vi "Generate_WayPoints_Hopping WITH VariablePauseTIME.vi"(11 "Input Cluster":T2={"Scan Rate (um/s)"=15.0, "X Start"=15.0, "X End"=15.0, "Y Start"=15.0, "Y End"=15.0, " Z Start"=15.0, "HoppingDistance"=1.0, "V"=15.0, "Z End"=15.0, "Approach Rate Hopping (um/s)"=15.0, "Retrack Rate (um/s)"=15.0, "V 2"=15.0, "Approach Rate (um/s)"=15.0, "Hold Time START / s"=15.0, "Hold Time Delta / s"=15.0, "Voltage to Electrode During Retract"=0.0, "Pause on First Approach?"=FALSE}) -> (1 "output cluster":T1)   [LabVIEW 2023]
uses:
  TypeDefs/WayPointCluster.ctl
panel:
  in  "WayPointCluster":T1
  out "Y  P":dbl
  out "X  P":dbl
  out "HoppingDistanceX":dbl
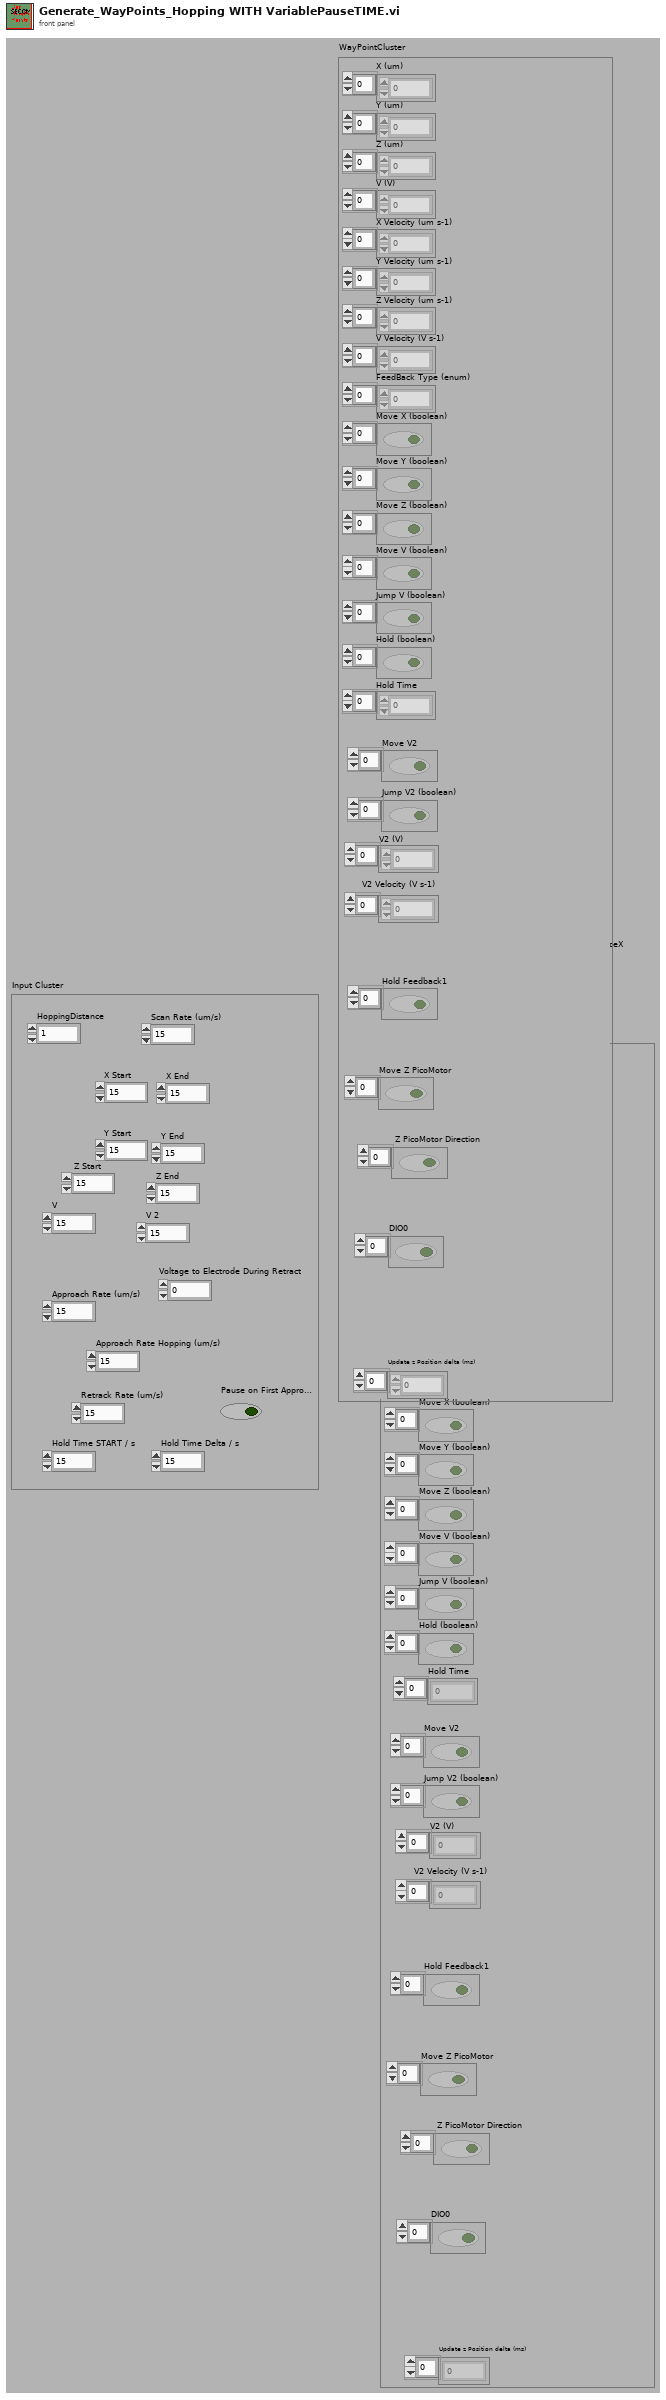
[diagram p1: front panel]
types:
  T1 = typedef "WayPointCluster.ctl" = cluster{"X (um)":dbl[], "Y (um)":dbl[], "Z (um)":dbl[], "V (V)":dbl[], "X Velocity (um s-1)":dbl[], "Y Velocity (um s-1)":dbl[], "Z Velocity (um s-1)":dbl[], "V Velocity (V s-1)":dbl[], "FeedBack Type (enum)":u16[], "Move X (boolean)":bool[], "Move Y (boolean)":bool[], "Move Z (boolean)":bool[], "Move V (boolean)":bool[], "Jump V (boolean)":bool[], "Hold (boolean)":bool[], "Hold Time":u32[], "V2 (V)":dbl[], "Move V2":bool[], "V2 Velocity (V s-1)":dbl[], "Jump V2 (boolean)":bool[], "Update z Position delta (ms)":i16[], "Hold Feedback1":bool[], "Move Z PicoMotor":bool[], " Z PicoMotor Direction":bool[], "DIO0":bool[]}
  T2 = cluster{"Scan Rate (um/s)":dbl, "X Start":dbl, "X End":dbl, "Y Start":dbl, "Y End":dbl, " Z Start":dbl, "HoppingDistance":dbl, "V":dbl, "Z End":dbl, "Approach Rate Hopping (um/s)":dbl, "Retrack Rate (um/s)":dbl, "V 2":dbl, "Approach Rate (um/s)":dbl, "Hold Time START / s":dbl, "Hold Time Delta / s":dbl, "Voltage to Electrode During Retract":dbl, "Pause on First Approach?":bool}
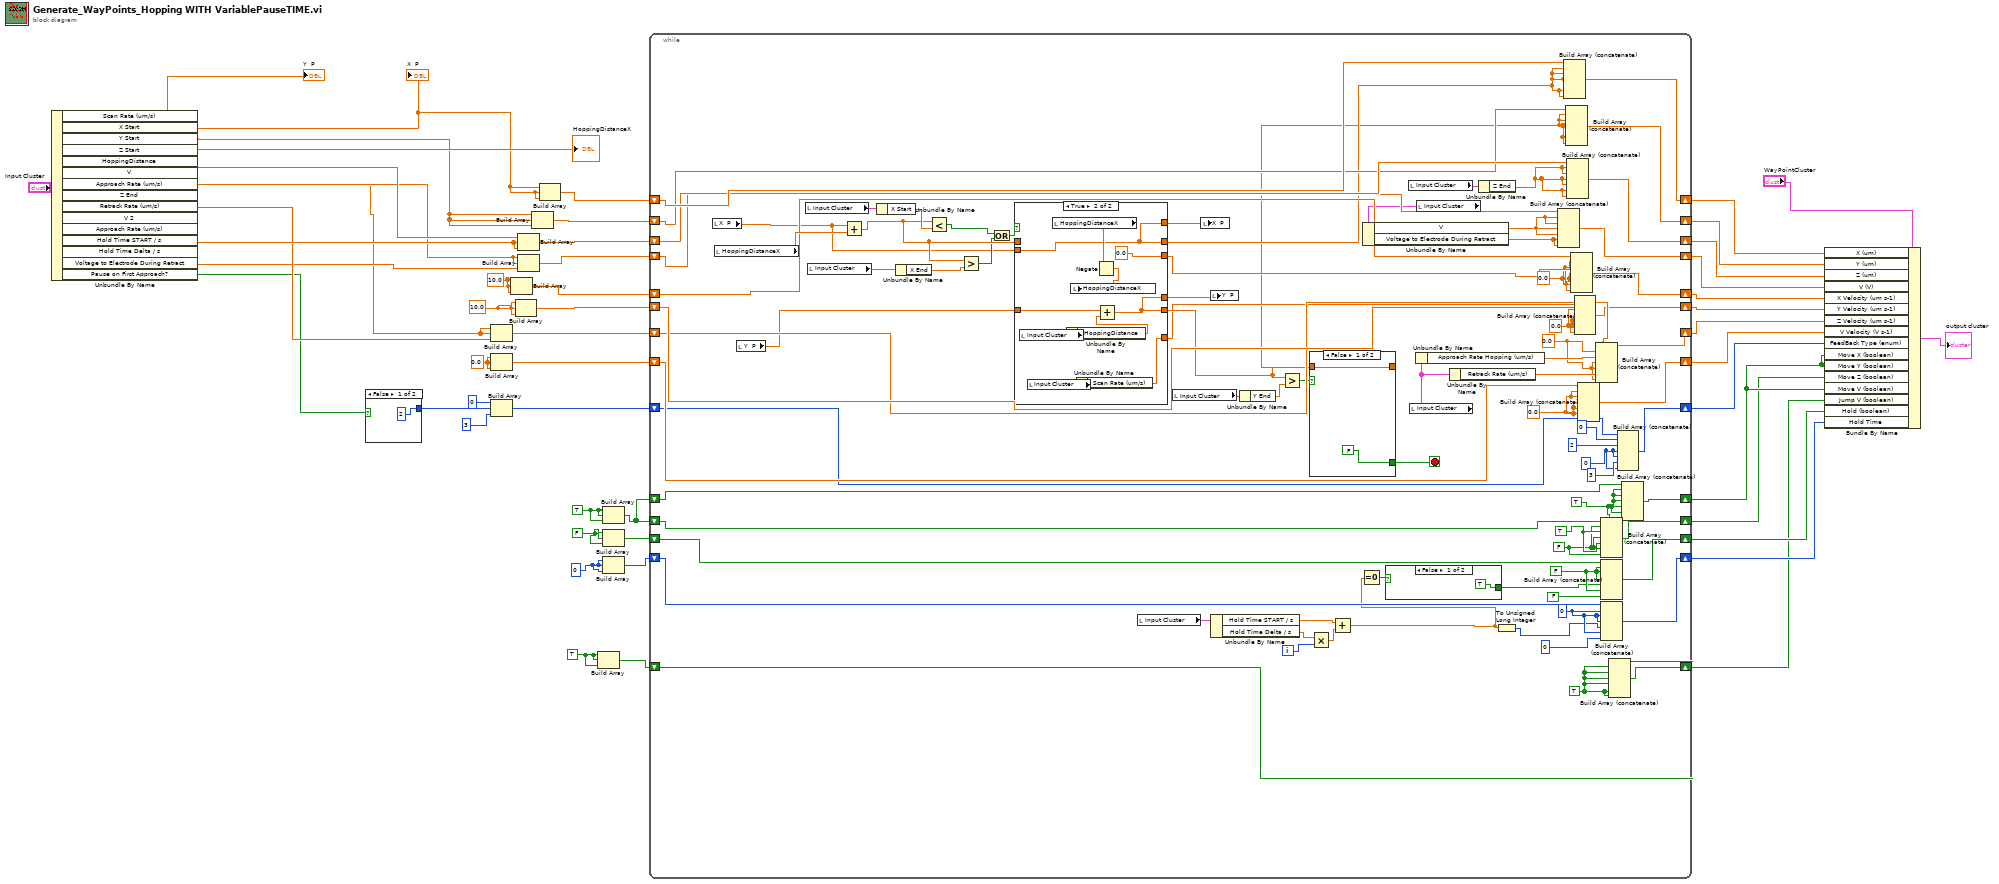
[diagram p0: block diagram]
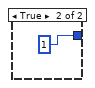
[diagram p2: hidden frame]
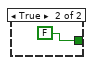
[diagram p3: hidden frame]
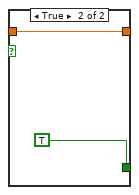
[diagram p4: hidden frame]
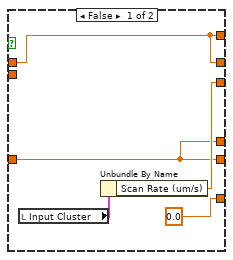
[diagram p5: hidden frame]
diagram:
  w11 = TRUE
  w12 = u32 0 ("element")
  w13 = FALSE
  w14 = TRUE
  w7 = 10.0 ("element")
  w8 = 10.0 ("element")
  w10 = 0.0 ("element")
  n1 = Unbundle By Name("Input Cluster") -> ("X Start"=w30:dbl, "Y Start"=w29:dbl, "Z Start"=w31:dbl, "HoppingDistance"=→"HoppingDistanceX":dbl, "V"=w27:dbl, "Approach Rate (um/s)"=w9:dbl, "Z End"=w28:dbl, "Retrack Rate (um/s)"=w26:dbl, "Voltage to Electrode During Retract"=w16:dbl, "Pause on First Approach?"=w4:bool)  [unwired: 5 out]
  "X  P" <- w30
  "Y  P" <- w29
  n2 = case shown="False" w4 {
    tunnel: [u16 2 ("element") u16 1 ("element")] -> w3
    frame False {
    }
    frame True {
    }
  }
  n3 = Build Array(w9, w9, w26) -> (w38:dbl[])
  n4 = Build Array(u16 0 ("element"), w3, u16 3 ("element")) -> (w34:u16[])
  n5 = Build Array(w10, w10, w10) -> (w36:dbl[])
  n6 = Build Array(w7, w7, w7) -> (w41:dbl[])
  n7 = Build Array(w8, w8, w8) -> (w40:dbl[])
  n8 = Build Array(w27, w27, w16) -> (w43:dbl[])
  n9 = Build Array(w31, w28, w28) -> (w45:dbl[])
  n10 = Build Array(w29, w29, w29) -> (w47:dbl[])
  n11 = Build Array(w30, w30, w30) -> (w49:dbl[])
  n12 = Build Array(w11, w11, w11) -> (w19:bool[])
  n13 = Build Array(w14, w14, w14) -> (w17:bool[])
  n14 = Build Array(w13, w13, w13) -> (w23:bool[])
  n15 = Build Array(w12, w12, w12) -> (w22:u32[])
  n16 = while {
    shift-right: [w131] -> w48
    shift-left: w49 -> [w132]
    shift-right: [w123] -> w46
    shift-left: w47 -> [w113]
    shift-right: [w122] -> w44
    shift-left: w45 -> [w130]
    shift-right: [w121] -> w42
    shift-left: w43 -> [w129]
    shift-right: [w120] -> w24
    shift-left: w41 -> [w128]
    shift-right: [w119] -> w39
    shift-left: w40 -> [w127]
    shift-right: [w118] -> w37
    shift-left: w38 -> [w126]
    shift-right: [w117] -> w35
    shift-left: w36 -> [w125]
    shift-right: [w116] -> w33
    shift-left: w34 -> [w124]
    shift-right: [w86] -> w1
    shift-left: w17 -> [w85]
    shift-right: [w87] -> w21
    shift-left: w23 -> [w91]
    shift-right: [w88] -> w20
    shift-left: w22 -> [w90]
    shift-right: [w83] -> w18
    shift-left: w19 -> [w84]
    shift-right: [w78] -> w2
    shift-left: w17 -> [w79]
    i -> [w80]
    stop <- w103 stop-if-true
    w59 = TRUE
    w55 = TRUE
    w72 = u32 0 ("element")
    w73 = FALSE
    w58 = FALSE
    w74 = TRUE
    w60 = u16 0 ("element")
    w63 = 0.0 ("element")
    w64 = 0.0 ("element")
    w61 = 0.0 ("element")
    w62 = 0.0 ("element")
    n17 = local read "X  P"() -> (w101:dbl)
    n18 = local read "HoppingDistanceX"() -> (w133:dbl)
    n19 = local read "Y  P"() -> (w100:dbl)
    n20 = local read "Input Cluster"() -> (w135:T2)
    n21 = local read "Input Cluster"() -> (w134:T2)
    n22 = Add(x=w101, y=w133) -> (x+y=w109:dbl)
    n23 = Unbundle By Name(w135) -> ("X Start"=w112:dbl)
    n24 = Unbundle By Name(w134) -> ("X End"=w110:dbl)
    n25 = Less?(x=w109, y=w112) -> (x < y?=w111:bool)
    n26 = Greater?(x=w109, y=w110) -> (0:w108:bool)
    n27 = Or(x=w111, y=w108) -> (x .or. y?=w107:bool)
    n28 = case shown="True" w107 {
      tunnel: w109 -> [w142 _]
      tunnel: [w142 w148] -> w68
      tunnel: w101 -> [_ w148]
      tunnel: w100 -> [w143 w149]
      tunnel: [w143 w147] -> w99
      tunnel: [w145 0.0] -> w93
      tunnel: [0.0 w150] -> w92
      tunnel: [w143 w147] -> w98
      tunnel: [w142 w148] -> w97
      frame False {
        n29 = local read "Input Cluster"() -> (w146:T2)
        n30 = Unbundle By Name(w146) -> ("Scan Rate (um/s)"=w145:dbl)
      }
      frame True {
        n31 = local read "Input Cluster"() -> (w154:T2)
        n32 = local read "Input Cluster"() -> (w152:T2)
        n33 = local read "HoppingDistanceX"() -> (w156:dbl)
        n34 = Unbundle By Name(w154) -> ("HoppingDistance"=w153:dbl)
        n35 = Unbundle By Name(w152) -> ("Scan Rate (um/s)"=w150:dbl)
        n36 = Negate(x=w156) -> (-x=w155:dbl)
        n37 = local write "HoppingDistanceX"(w155) -> ()
        n38 = Add(x=w149, y=w153) -> (x+y=w147:dbl)
      }
    }
    n39 = local read "Input Cluster"() -> (w89:T2)
    n40 = local read "Input Cluster"() -> (w106:T2)
    n41 = local write "X  P"(w97) -> ()
    n42 = local write "Y  P"(w98) -> ()
    n43 = Unbundle By Name(w89) -> ("Hold Time START / s"=w69:dbl, "Hold Time Delta / s"=w82:dbl)
    n44 = Unbundle By Name(w106) -> ("Y End"=w105:dbl)
    n45 = Greater?(x=w99, y=w105) -> (0:w104:bool)
    n46 = case shown="False" w104 {
      tunnel: w99 -> [w139 w141]
      tunnel: [w139 w141] -> w67
      tunnel: [FALSE TRUE] -> w103
      frame False {
      }
      frame True {
      }
    }
    n47 = Multiply(x=w82, y=w80) -> (x*y=w81:dbl)
    n48 = Add(x=w69, y=w81) -> (x+y=w54:dbl)
    n49 = Equal To 0?(x=w54) -> (x = 0?=w70:bool)
    n50 = case shown="False" w70 {
      tunnel: [TRUE FALSE] -> w71
      frame False {
      }
      frame True {
      }
    }
    n51 = local read "Input Cluster"() -> (w115:T2)
    n52 = local read "Input Cluster"() -> (w102:T2)
    n53 = Unbundle By Name(w102) -> ("Approach Rate Hopping (um/s)"=w94:dbl)
    n54 = local read "Input Cluster"() -> (w114:T2)
    n55 = Unbundle By Name(w114) -> ("V"=w77:dbl, "Voltage to Electrode During Retract"=w65:dbl)
    n56 = Unbundle By Name(w102) -> ("Retrack Rate (um/s)"=w76:dbl)
    n57 = Unbundle By Name(w115) -> ("Z End"=w66:dbl)
    n58 = To Unsigned Long Integer(number=w54) -> (unsigned 32bit integer=w53:u32)
    n59 = Build Array (concatenate)(w129, w77, w77, w77, w77, w65, w65) -> (w121:dbl[])
    n60 = Build Array (concatenate)(w132, w68, w68, w68, w68, w68, w68) -> (w131:dbl[])
    n61 = Build Array (concatenate)(w113, w67, w67, w67, w67, w67, w67) -> (w123:dbl[])
    n62 = Build Array (concatenate)(w130, w66, w66, w66, w66, w66, w66) -> (w122:dbl[])
    n63 = Build Array (concatenate)(w128, w93, w64, w64, w64, w64, w64) -> (w120:dbl[])
    n64 = Build Array (concatenate)(w127, w92, w63, w63, w63, w63, w63) -> (w119:dbl[])
    n65 = Build Array (concatenate)(w125, w61, w61, w61, w61, w61, w61) -> (w117:dbl[])
    n66 = Build Array (concatenate)(w126, w62, w94, w62, w62, w76, w62) -> (w118:dbl[])
    n67 = Build Array (concatenate)(w85, w58, w74, w58, w58, w74, w58) -> (w86:bool[])
    n68 = Build Array (concatenate)(w91, w73, w73, w73, w71, w73, FALSE ("element")) -> (w87:bool[])
    n69 = Build Array (concatenate)(w90, w72, w72, w72, w53, w72, u32 0 ("element")) -> (w88:u32[])
    n70 = Build Array (concatenate)(w84, w55, w55, w55, w55, w55, w55) -> (w83:bool[])
    n71 = Build Array (concatenate)(w124, u16 0 ("element"), u16 2 ("element"), w60, w60, u16 3 ("element"), w60) -> (w116:u16[])
    n72 = Build Array (concatenate)(w79, w59, w59, w59, w59, w59, w59) -> (w78:bool[])
  }
  n73 = Bundle By Name(cluster="WayPointCluster", "X (um)"=w48, "Y (um)"=w46, "Z (um)"=w44, "V (V)"=w42, "X Velocity (um s-1)"=w24, "Y Velocity (um s-1)"=w39, "Z Velocity (um s-1)"=w37, "V Velocity (V s-1)"=w35, "FeedBack Type (enum)"=w33, "Move X (boolean)"=w2, "Move Y (boolean)"=w2, "Move Z (boolean)"=w1, "Move V (boolean)"=w2, "Jump V (boolean)"=w18, "Hold (boolean)"=w21, "Hold Time"=w20) -> (→"output cluster":T1)
